vi "setFunction.vi"(8 "error in (no error)":errorcluster, 10 "Function":u8, 11 "FrameBuilder in":refnum<class "FrameBuilder.lvclass">) -> (0 "error out":errorcluster, 3 "FrameBuilder out":refnum<class "FrameBuilder.lvclass">)   [LabVIEW 2015, in "FrameBuilder.lvclass"]
uses:
  FrameBuilder.lvclass
  FrameBuilder.lvclass/FrameBuilder.ctl
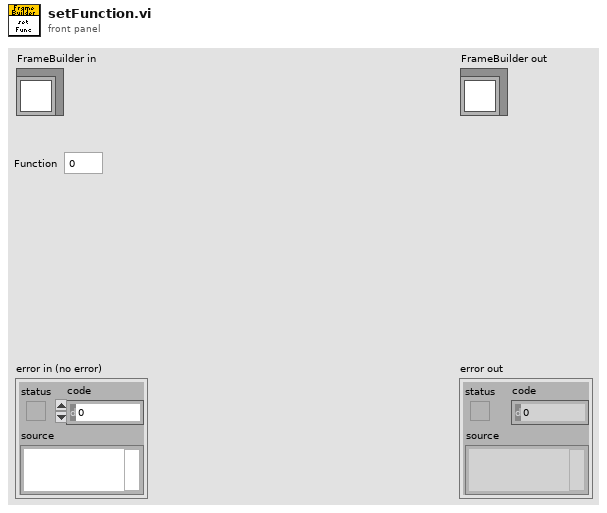
[diagram p1: front panel]
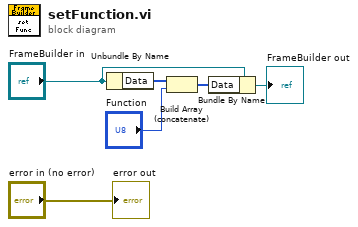
[diagram p0: block diagram]
diagram:
  n1 = Unbundle By Name("FrameBuilder in") -> ("Data"=w5:u8[])
  n2 = Build Array (concatenate)(w5, "Function") -> (w3:u8[])
  n3 = Bundle By Name(cluster="FrameBuilder in", "Data"=w3) -> (→"FrameBuilder out":refnum<class "FrameBuilder.lvclass">)
  "error out" <- "error in (no error)"
